vi "Wrap Message.vi"(7 "Sender":string, 8 "error in (no error)":errorcluster, 9 "Data":variant, 10 "Message":string, 11 "Recipient":string) -> (0 "error out":errorcluster, 3 "Message out":refnum<class "Message.lvclass">)   [LabVIEW 2018, in "Application.lvlib" / "Message.lvclass"]
uses:
  Message.lvclass
  Message.lvclass/Message.ctl
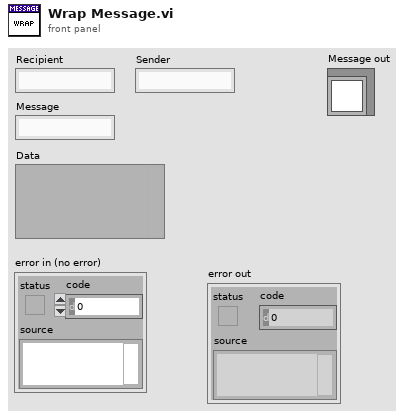
[diagram p1: front panel]
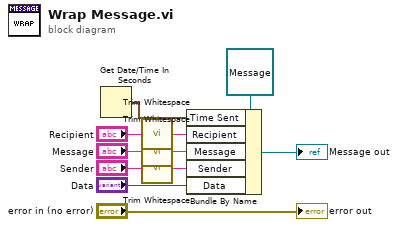
[diagram p0: block diagram]
diagram:
  n1 = Get Date/Time In Seconds() -> (seconds since 1Jan1904=w7:timestamp)
  n2 = call <vilib>:"Trim Whitespace.vi"("string"="Recipient") -> ("trimmed string"=w3:string)  [unwired: 1 in]
  n3 = call <vilib>:"Trim Whitespace.vi"("string"="Message") -> ("trimmed string"=w2:string)  [unwired: 1 in]
  n4 = call <vilib>:"Trim Whitespace.vi"("string"="Sender") -> ("trimmed string"=w1:string)  [unwired: 1 in]
  n5 = Bundle By Name(cluster=refnum<class "Message.lvclass"> refnum ("Message in"), "Time Sent"=w7, "Recipient"=w3, "Message"=w2, "Sender"=w1, "Data"="Data") -> (→"Message out":refnum<class "Message.lvclass">)
  "error out" <- "error in (no error)"
